vi "Asana_Post.vi"() -> ()   [LabVIEW 2016]
uses:
  <vilib>/httpClient/POSTBuffer.vi
  <vilib>/httpClient/LabVIEWHTTPClient.lvlib
panel:
  out "Status":string="Standing by"
  out "HTTP Returned Body":string="{\"data\":{\"id\":485255656454849,\"created_at\":\"2017-11-21T16:39:33.429Z\",\"modified_at\":\"2017-11-21T16:39:33.429Z\",\"name\":\"Figure out useful API\",\"notes\":\"Separator is 'and' sign.\",\"assignee\":{\"id\":15435307170131,\"name\":\"Yun-Yi Pai\"},\"completed\":false,\"assignee_status\":\"inbox\",\"completed_at\":null,\"due_on\":null,\"due_at\":null,\"projects\":[],\"memberships\":[],\"tags\":[],\"workspace\":{\"id\":914676468468,\"name\":\"levylab.org\"},\"num_hearts\":0,\"parent\":null,\"hearted\":false,\"hearts\":[],\"custom_fields\":[],\"followers\":[{\"id\":15435307170131,\"name\":\"Yun-Yi Pai\"}]}}"
  out "HTTP Returned Headers":string="HTTP/1.1 201 Created\r\nServer: nginx\r\nDate: Tue, 21 Nov 2017 16:39:34 GMT\r\nContent-Type: application/json; charset=UTF-8\r\nTransfer-Encoding: chunked\r\nConnection: keep-alive\r\nCache-Control: no-store\r\nPragma: no-cache\r\nLocation: /api/1.0/tasks/485255656454849\r\nX-Asana-Content-String-Length: 549\r\nSet-Cookie: TooBusyRedirectCount=0\r\nX-Server-Name: prod-ws022.ec2\r\nX-Asana-Preferred-Release-Revision: 20171120_221241_867ba3e15db2221bfc1a505ff00d5822edf28beb\r\nX-Asana-Api-Version: 1.0\r\nX-Robots-Tag: none\r\nStrict-Transport-Security: max-age=31536000; includeSubDomains\r\nDatacenter-Time-End: 1511282374.035\r\nX-LoadBalancer: prod-lb000.ec2\r\n\r\n"
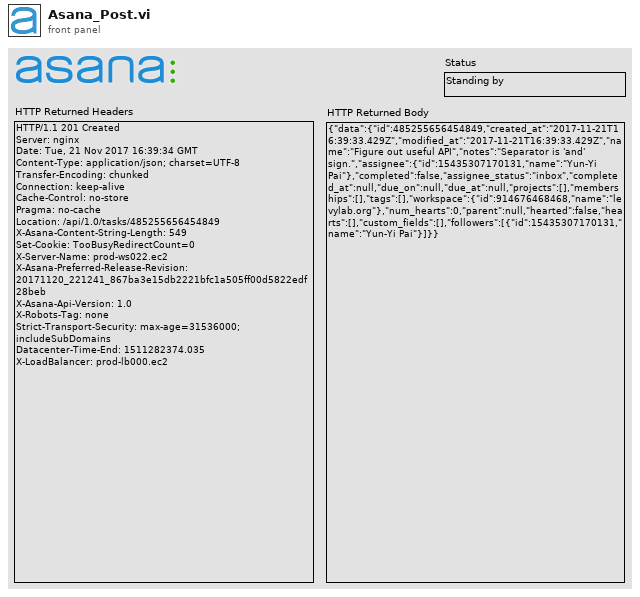
[diagram p1: front panel]
types:
  T1 = typedef "LabVIEWHTTPClient.lvlib/ClientHandle.ctl" = refnum<k1>
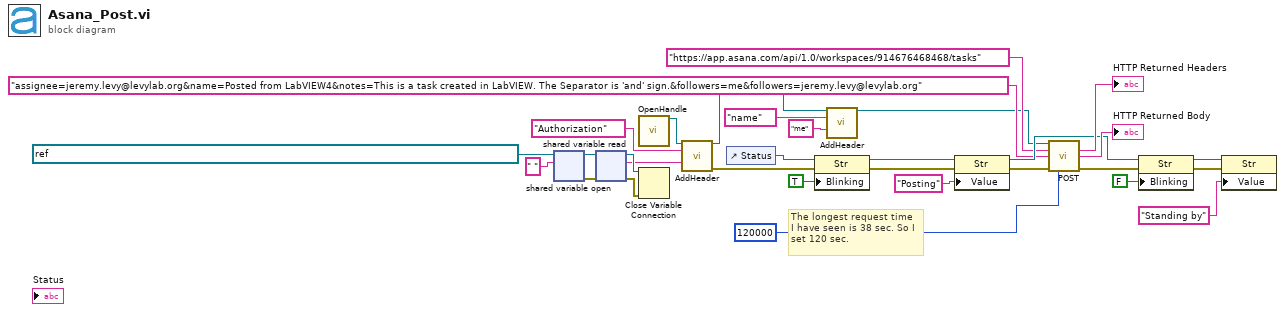
[diagram p0: block diagram]
diagram:
  # "The longest request time\nI have seen is 38 sec. So I\nset 120 sec."
  n1 = shared-variable-open(refnum<k21> "ni.var.psp://housesoftheholy/OneNote API HTTP/Asana Access Token 15669051163913" ("shared variable refnum in"), " " ("string")) -> (w25:refnum<k21>, w24:errorcluster)  [unwired: 2 in]
  n2 = shared-variable-read(w25, w24) -> (w22:refnum<k21>, w23:errorcluster, w21:string)  [unwired: 1 out]
  n3 = call <vilib>:"OpenHandle.vi"() -> ("client handle out"=w29:T1)  [unwired: 14 in, 1 out]
  n4 = Close Variable Connection(8:w23, 11:w22) -> ()  [unwired: 1 out]
  n5 = call <vilib>:"AddHeader.vi"("client handle"=w29, "header"="Authorization", "value"=w21) -> ("client handle out"=w2:T1, "error out"=w6:errorcluster)  [unwired: 11 in]
  n6 = control-ref of="Status"() -> (w14:refnum<vi>)
  n7 = property on="Property Node" class="Str"(reference=w14, error in=w6, "Blinking"=TRUE) -> (reference out=w13:refnum<vi>, error out=w12:errorcluster)
  n8 = call <vilib>:"AddHeader.vi"("client handle"=w2, "header"="name", "value"="me") -> ("client handle out"=w1:T1)  [unwired: 11 in, 1 out]
  n9 = property on="Property Node" class="Str"(reference=w13, error in=w12, "Value"="Posting" ("Status")) -> (reference out=w10:refnum<vi>, error out=w11:errorcluster)
  n10 = call-poly <vilib>:"POST.vi"("client handle"=w1, "url"="https://app.asana.com/api/1.0/workspaces/914676468468/tasks", "buffer"="assignee=jeremy.levy@levylab.org&name=Posted from LabVIEW4&notes=This is a task created in LabVIEW. The Separator is 'and' sign.&followers=me&followers=jeremy.levy@levylab.org", "error in (no error)"=w11, "timeout (10000)"=120000) -> ("headers"=→"HTTP Returned Headers":string, "body"=→"HTTP Returned Body":string, "error out"=w9:errorcluster)  [unwired: 7 in, 1 out]
  n11 = property on="Property Node" class="Str"(reference=w10, error in=w9, "Blinking"=FALSE ("Visible")) -> (reference out=w8:refnum<vi>, error out=w15:errorcluster)
  n12 = property on="Property Node" class="Str"(reference=w8, error in=w15, "Value"="Standing by" ("Status")) -> ()  [unwired: 2 out]
